vi "3motorVelCtrlTest.vi"() -> ()   [LabVIEW 2020]
uses:
  <vilib>/Platform/TimedLoop/XDataNode/timing_clust.ctl
  <vilib>/Platform/TimedLoop/XDataNode/nitl_modes.ctl
  <vilib>/Platform/TimedLoop/XDataNode/wakeup.ctl
  <vilib>/CISH Robotics/L4VMX TitanQuad/Motor ID.ctl
  <vilib>/CISH Robotics/L4VMX TitanQuad/TitanQuad.lvclass
  <vilib>/platform/TimedLoop/XDataNode/XDataNode.xnode
  <vilib>/Platform/TimedLoop/XDataNode/XDNodeRunTimeDep.lvlib
panel:
  out "error out":errorcluster
  out "Enc [M0, M1, M2] (deg)":dbl[](array[numeric])
  in  "error in (no error)":errorcluster
  out "Finished Late? [i-1]":bool
  in  "reset Encoder":bool
  in  "Stop Button":bool
  in  "motorSpeed [M0, M1, M2] (deg/s)":dbl[](array[slide]) scale=-450.0..450.0
  # "M0-M2 「左、右、後輪」 正轉逆時針\nM3 正轉爪向上"
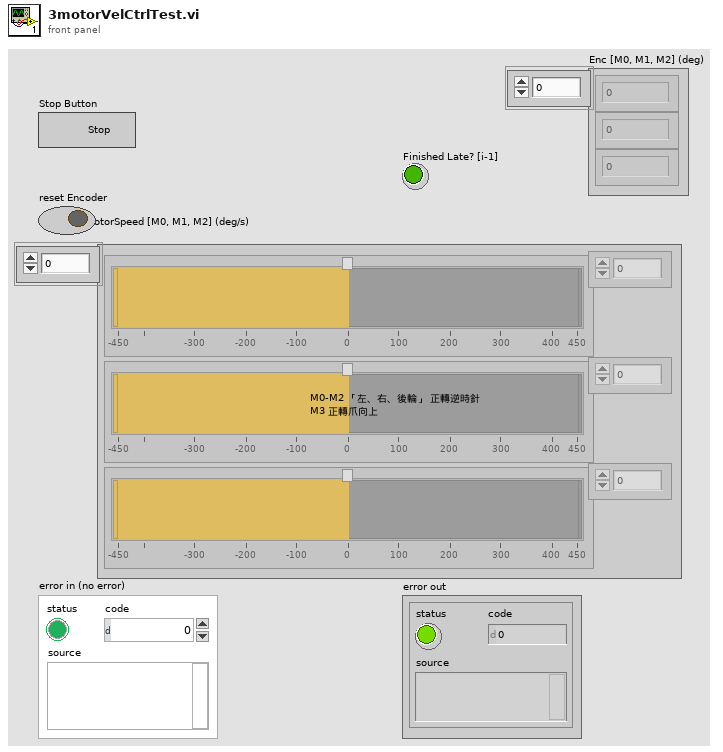
[diagram p1: front panel]
types:
  T1 = typedef "TitanQuad.lvlib/TitanQuad.lvclass/Motor ID.ctl" = enum16{"M0", "M1", "M2", "M3"}
  T2 = typedef "XDNodeRunTimeDep.lvlib/timing_clust.ctl" = cluster{"Expected End [f-1]":u64, "Actual End [f-1]":u64, "Finished Late? [f-1]":bool, "Expected End [i-1]":u64, "Actual End [i-1]":u64, "Finished Late? [i-1]":bool, "Expected Start [i]":u64, "Actual Start [i]":u64, "Expected Start [f]":u64, "Actual Start [f]":u64, "Source Name":string, "Structure Name":string, "Period":i64, "Deadline":i64, "Offset":i64, "Start":i64, "Priority":i32, "Timeout":i32, "Mode":T3, "Wakeup Reason":T4, "Error":errorcluster, "Source Type":string, "Secondary Source Type":string, "Global End Time":u64, "Global Start Time":u64, "Frame Duration":u64, "Iteration Duration":u64, "Assigned CPU":i32, "I/O Scan Engine Mode":u32}
  T3 = typedef "XDNodeRunTimeDep.lvlib/nitl_modes.ctl" = enum32{"No Change", "Process missed periods, maintain original phase", "Discard missed periods, maintain original phase", "Process missed periods, ignore original phase", "Discard missed periods, ignore original phase"}
  T4 = typedef "XDNodeRunTimeDep.lvlib/wakeup.ctl" = enum32{"Normal", "Aborted", "Asynchronous wakeup", "Timing source error", "Timed loop error", "Timeout"}
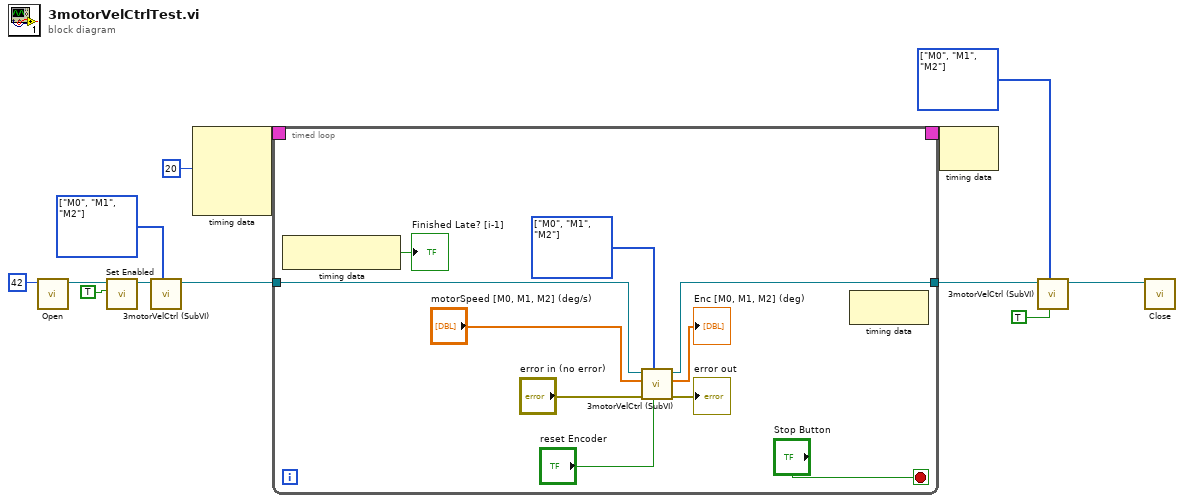
[diagram p0: block diagram]
diagram:
  w2 = T1[] [enum."M0", enum."M1", enum."M2"] items=["M0", "M1", "M2", "M3"] ("motorPort [M0, M1, M2]")
  w3 = T1[] [enum."M0", enum."M1", enum."M2"] items=["M0", "M1", "M2", "M3"] ("motorPort [M0, M1, M2]")
  n1 = call <vilib>:"Open.vi"("Titan ID (42)"=u8 42) -> ("TitanQuad Object"=w13:refnum<class "TitanQuad.lvclass">)  [unwired: 9 in, 1 out]
  n2 = call <vilib>:"Set Enabled.vi"("Enable"=TRUE, "TitanQuad Object"=w13) -> ("TitanQuad Object"=w5:refnum<class "TitanQuad.lvclass">)  [unwired: 8 in, 1 out]
  n3 = call "3motorVelCtrl (SubVI).vi"("motorPort [M0, M1, M2]"=w3, "TitanQuad in"=w5) -> ("TitanQuad out"=w4:refnum<class "TitanQuad.lvclass">)  [unwired: 7 in, 2 out]
  n4 = node-c288(i64 20 ("Period")) -> (w10:T2)  [unwired: 3 in]
  n5 = timed-loop {
    tunnel: w4 -> [w20]
    tunnel: [w23] -> w7
    timing: w10 -> [_]
    timing-out: [_] -> w9
    stop <- "Stop Button" stop-if-true
    w14 = T1[] [enum."M0", enum."M1", enum."M2"] items=["M0", "M1", "M2", "M3"] ("motorPort [M0, M1, M2]")
    n6 = node-c288() -> (→"Finished Late? [i-1]":bool)  [unwired: 1 in]
    n7 = call "3motorVelCtrl (SubVI).vi"("reset Encoder"="reset Encoder", "motorPort [M0, M1, M2]"=w14, "error in (no error)"="error in (no error)", "motorSpeed [M0, M1, M2] (deg/s)"="motorSpeed [M0, M1, M2] (deg/s)", "TitanQuad in"=w20) -> ("error out"=→"error out":errorcluster, "Enc [M0, M1, M2] (deg)"=→"Enc [M0, M1, M2] (deg)":dbl[], "TitanQuad out"=w23:refnum<class "TitanQuad.lvclass">)  [unwired: 4 in]
    n8 = node-c288() -> ()  [unwired: 1 in, 1 out]
  }
  n9 = node-c288(w9) -> ()  [unwired: 1 out]
  n10 = call "3motorVelCtrl (SubVI).vi"("reset Encoder"=TRUE, "motorPort [M0, M1, M2]"=w2, "TitanQuad in"=w7) -> ("TitanQuad out"=w1:refnum<class "TitanQuad.lvclass">)  [unwired: 6 in, 2 out]
  n11 = call <vilib>:"Close.vi"("TitanQuad Object"=w1) -> ()  [unwired: 10 in, 1 out]
